vi "LvMPDC_SUB_ParseReplyString_Status.vi"(10 "status reply string":string="volume: 90\nrepeat: 0\nrandom: 0\nsingle: 0\nconsume: 1\nplaylist: 10\nplaylistlength: 6\nxfade: 0\nmixrampdb: 0.000000\nmixrampdelay: nan\nstate: play\nsong: 0\nsongid: 8\ntime: 48:264\nelapsed: 47.833\nbitrate: 128\naudio: 22050:24:1\nnextsong: 1\nnextsongid: 9\n") -> (2 "status":T1 {"elapsed" format="%<%H:%M:%S%3u>t"; "time" format="%<%H:%M:%S%3u>t"})   [LabVIEW 2012]
uses:
  LvMPDC_Typdef_status.ctl
panel:
  # "volume: 90\nrepeat: 0\nrandom: 0\nsingle: 0\nconsume: 1\nplaylist: 10\nplaylistlength: 6\nxfade: 0[sec]\nmixrampdb: 0.000000\nmixrampdelay: nan\nstate: play\nsong: 0\nsongid: 8\ntime: 48:264\nelapsed: 47.833\nbitrate: 128[kbps]\naudio: 22050:24:1\nnextsong: 1\nnextsongid: 9"
  # "volume: 90\nrepeat: 0\nrandom: 0\nsingle: 0\nconsume: 1\nplaylist: 16\nplaylistlength: 0\nxfade: 0\nmixrampdb: 0.000000[dB]\nmixrampdelay: nan[sec]\nstate: stop"
  # "audio: 22050:24:1 / samplerate:bits:channels"
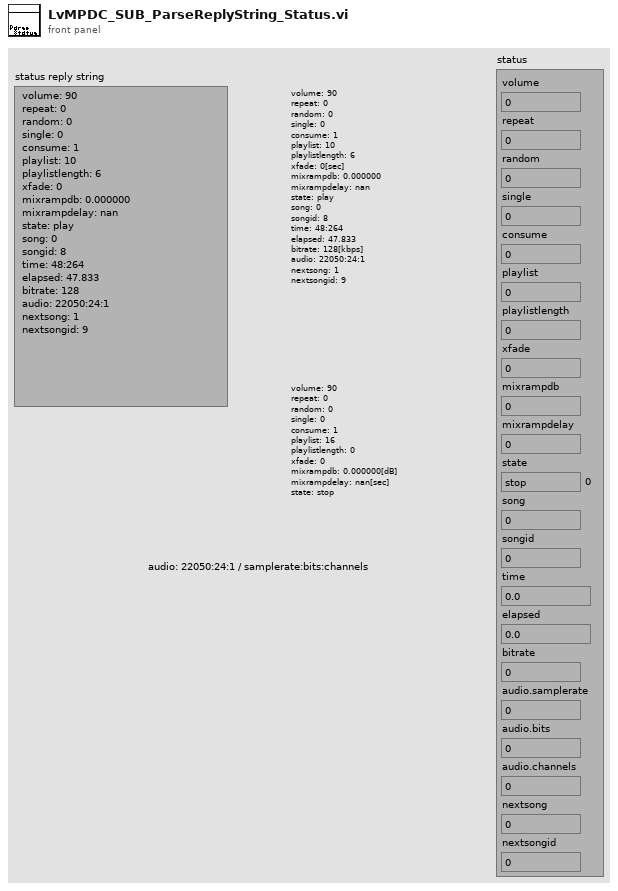
[diagram p1: front panel]
types:
  T1 = typedef "LvMPDC_Typdef_status.ctl" = cluster{"volume":i32, "repeat":i32, "random":i32, "single":i32, "consume":i32, "playlist":i32, "playlistlength":i32, "xfade":i32, "mixrampdb":dbl, "mixrampdelay":dbl, "state":enum16{"stop", "play", "pause"}, "song":i32, "songid":i32, "time":dbl, "elapsed":dbl, "bitrate":i32, "audio.samplerate":i32, "audio.bits":i32, "audio.channels":i32, "nextsong":i32, "nextsongid":i32}
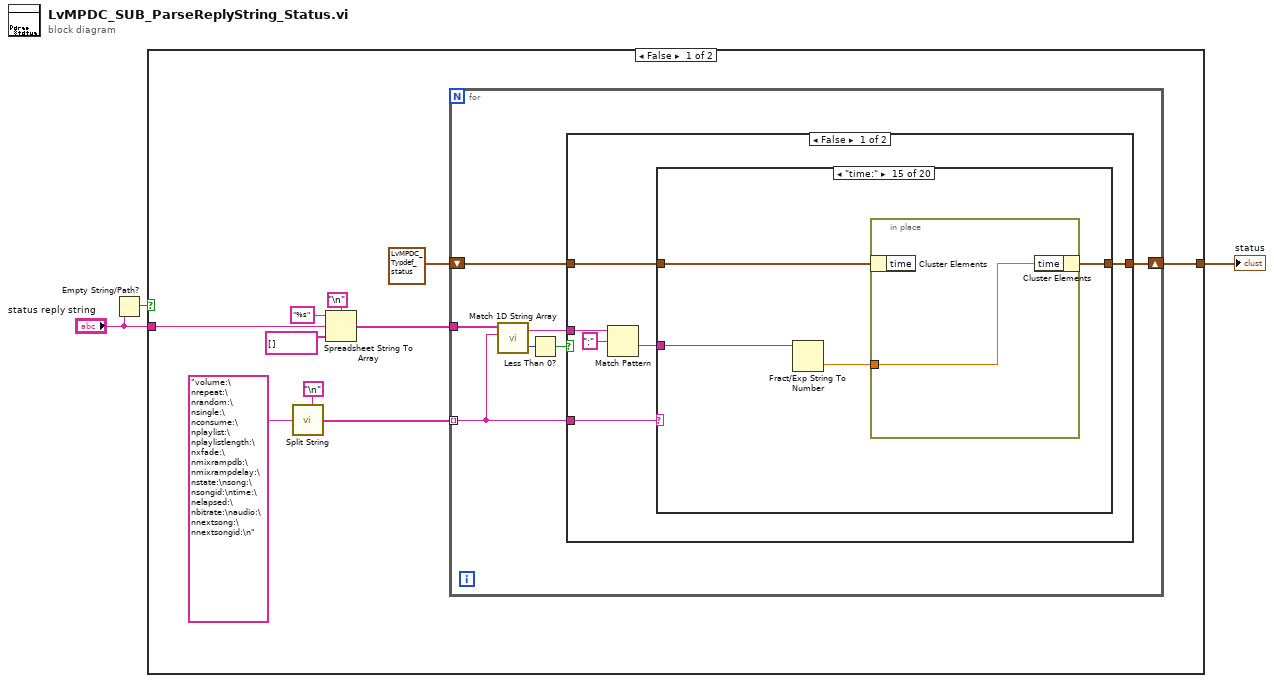
[diagram p0: block diagram]
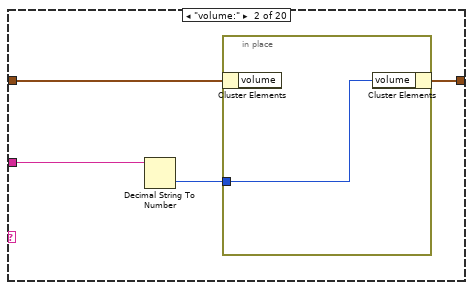
[diagram p3: hidden frame]
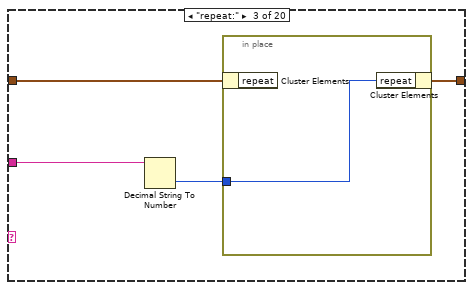
[diagram p4: hidden frame]
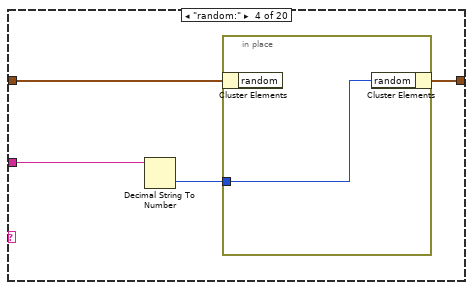
[diagram p5: hidden frame]
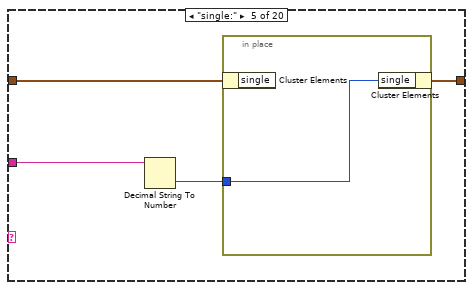
[diagram p6: hidden frame]
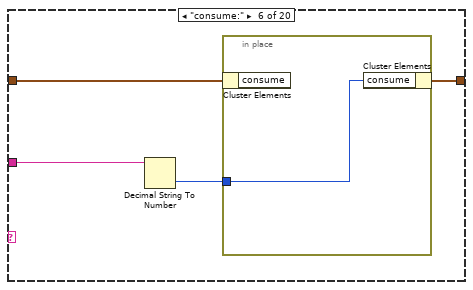
[diagram p7: hidden frame]
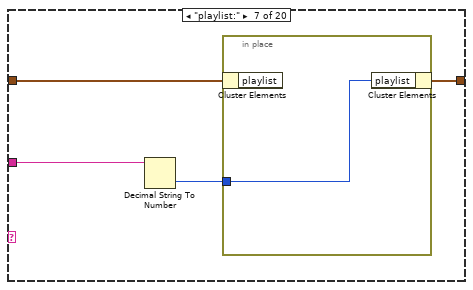
[diagram p8: hidden frame]
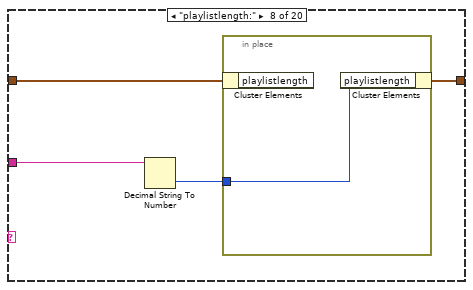
[diagram p9: hidden frame]
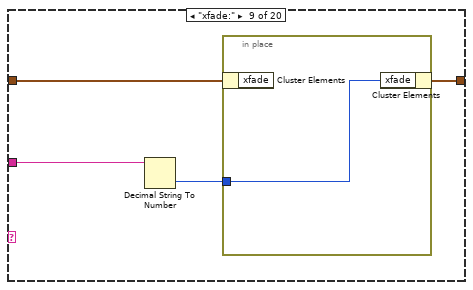
[diagram p10: hidden frame]
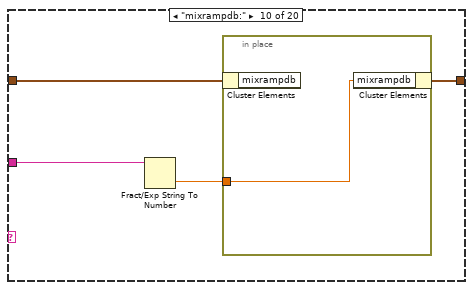
[diagram p11: hidden frame]
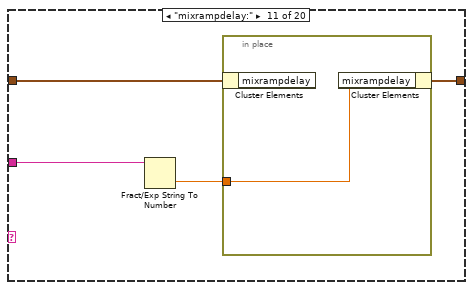
[diagram p12: hidden frame]
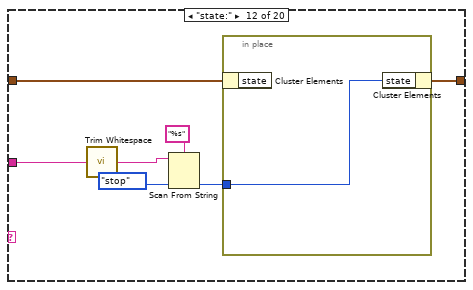
[diagram p13: hidden frame]
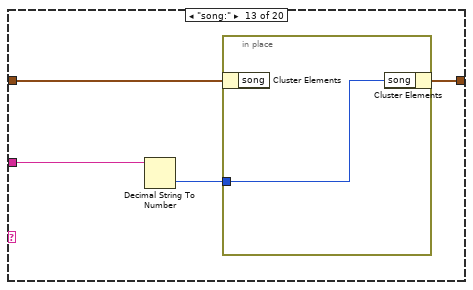
[diagram p14: hidden frame]
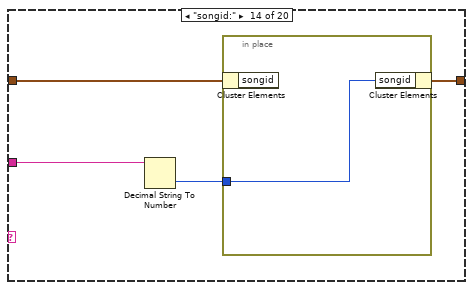
[diagram p15: hidden frame]
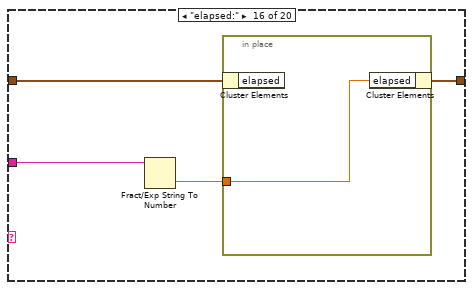
[diagram p16: hidden frame]
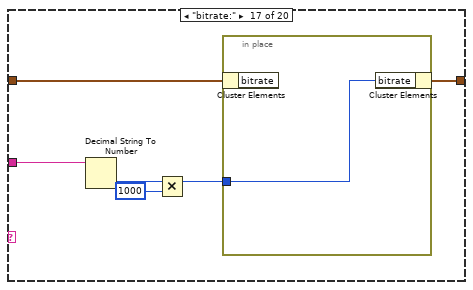
[diagram p17: hidden frame]
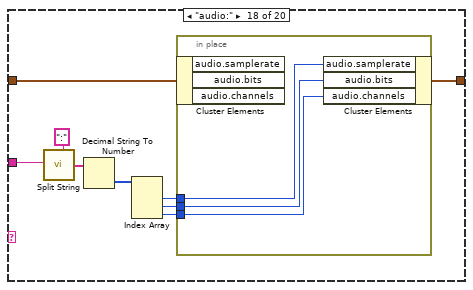
[diagram p18: hidden frame]
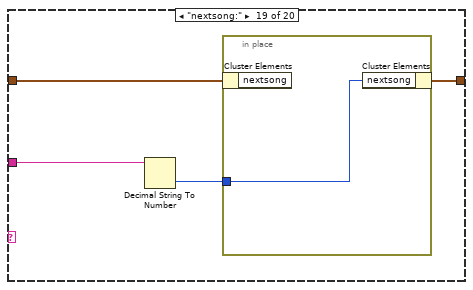
[diagram p19: hidden frame]
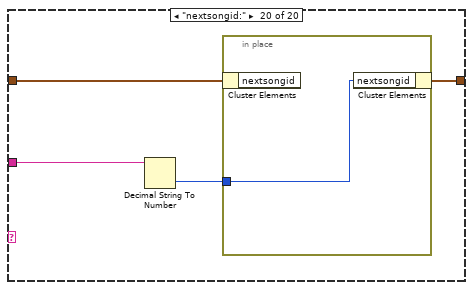
[diagram p20: hidden frame]
diagram:
  n1 = Empty String/Path?(string/path="status reply string") -> (empty?=w1:bool)
  n2 = case shown="FALSE" w1 {
    tunnel: "status reply string" -> [w10 _]
    tunnel: [w5 _] -> w3
    frame False {
      n3 = call <vilib>:"Split String.vi"("Split Pattern"="\n", "Input String"="volume:\nrepeat:\nrandom:\nsingle:\nconsume:\nplaylist:\nplaylistlength:\nxfade:\nmixrampdb:\nmixrampdelay:\nstate:\nsong:\nsongid:\ntime:\nelapsed:\nbitrate:\naudio:\nnextsong:\nnextsongid:\n") -> ("Split String"=w6:string[])  [unwired: 5 in]
      n4 = Spreadsheet String To Array(delimiter (Tab)="\n", format string="%s" ("形式文字列"), spreadsheet string=w10, array type (2D Dbl)=string[] []) -> (array=w9:string[])
      n5 = for {
        tunnel: w9 -> [w20]
        tunnel: w6 -> [w19] mode=indexing
        shift-right: [w14] -> w5
        shift-left: T1 {"volume"=0, "repeat"=0, "random"=0, "single"=0, "consume"=0, "playlist"=0, "playlistlength"=0, "xfade"=0, "mixrampdb"=0.0, "mixrampdelay"=0.0, "state"=enum."stop", "song"=0, "songid"=0, "time"=0.0, "elapsed"=0.0, "bitrate"=0, "audio.samplerate"=0, "audio.bits"=0, "audio.channels"=0, "nextsong"=0, "nextsongid"=0} ("status") -> [w15]
        n6 = call <vilib>:"Match 1D String Array.vi"("Pattern"=w19, "Strings"=w20) -> ("index of element"=w18:i32, "Match"=w17:string)  [unwired: 2 in]
        n7 = Less Than 0?(x=w18) -> (x < 0?=w16:bool)
        n8 = case shown="FALSE" w16 {
          tunnel: w19 -> [w26 _]
          tunnel: w17 -> [w22 _]
          tunnel: w15 -> [w25 w135]
          tunnel: [w24 w135] -> w14
          frame False {
            n9 = Match Pattern(string=w22, regular expression=":" ("正規表現")) -> (after substring=w21:string)  [unwired: 1 in, 3 out]
            n10 = case shown="\"time:\"" w26 {
              tunnel: w25 -> [w27 w31 w36 w41 w46 w51 w56 w61 w66 w71 w76 w84 w89 w94 w99 w104 w111 w121 w128 w133]
              tunnel: [w27 w30 w35 w40 w45 w50 w55 w60 w65 w70 w75 w83 w88 w93 w98 w103 w110 w120 w127 w132] -> w24
              tunnel: w21 -> [_ w29 w34 w39 w44 w49 w54 w59 w64 w69 w74 w82 w87 w92 w97 w102 w109 w119 w126 w131]
              frame Default {
              }
              frame "volume:" {
                n11 = Decimal String To Number(string=w29) -> (number=w28:i32)  [unwired: 2 in, 1 out]
                n12 = in-place {
                  in-place-border: w28 -> [w32]
                  n13 = in-place-cluster #1(w31) -> ()  [unwired: 1 out]
                  n14 = in-place-cluster #1("volume"=w32) -> (w30:T1)
                }
              }
              frame "repeat:" {
                n15 = Decimal String To Number(string=w34) -> (number=w33:i32)  [unwired: 2 in, 1 out]
                n16 = in-place {
                  in-place-border: w33 -> [w37]
                  n17 = in-place-cluster #2(w36) -> ()  [unwired: 1 out]
                  n18 = in-place-cluster #2("repeat"=w37) -> (w35:T1)
                }
              }
              frame "random:" {
                n19 = Decimal String To Number(string=w39) -> (number=w38:i32)  [unwired: 2 in, 1 out]
                n20 = in-place {
                  in-place-border: w38 -> [w42]
                  n21 = in-place-cluster #3(w41) -> ()  [unwired: 1 out]
                  n22 = in-place-cluster #3("random"=w42) -> (w40:T1)
                }
              }
              frame "single:" {
                n23 = Decimal String To Number(string=w44) -> (number=w43:i32)  [unwired: 2 in, 1 out]
                n24 = in-place {
                  in-place-border: w43 -> [w47]
                  n25 = in-place-cluster #4(w46) -> ()  [unwired: 1 out]
                  n26 = in-place-cluster #4("single"=w47) -> (w45:T1)
                }
              }
              frame "consume:" {
                n27 = Decimal String To Number(string=w49) -> (number=w48:i32)  [unwired: 2 in, 1 out]
                n28 = in-place {
                  in-place-border: w48 -> [w52]
                  n29 = in-place-cluster #5(w51) -> ()  [unwired: 1 out]
                  n30 = in-place-cluster #5("consume"=w52) -> (w50:T1)
                }
              }
              frame "playlist:" {
                n31 = Decimal String To Number(string=w54) -> (number=w53:i32)  [unwired: 2 in, 1 out]
                n32 = in-place {
                  in-place-border: w53 -> [w57]
                  n33 = in-place-cluster #6(w56) -> ()  [unwired: 1 out]
                  n34 = in-place-cluster #6("playlist"=w57) -> (w55:T1)
                }
              }
              frame "playlistlength:" {
                n35 = Decimal String To Number(string=w59) -> (number=w58:i32)  [unwired: 2 in, 1 out]
                n36 = in-place {
                  in-place-border: w58 -> [w62]
                  n37 = in-place-cluster #7(w61) -> ()  [unwired: 1 out]
                  n38 = in-place-cluster #7("playlistlength"=w62) -> (w60:T1)
                }
              }
              frame "xfade:" {
                n39 = Decimal String To Number(string=w64) -> (number=w63:i32)  [unwired: 2 in, 1 out]
                n40 = in-place {
                  in-place-border: w63 -> [w67]
                  n41 = in-place-cluster #8(w66) -> ()  [unwired: 1 out]
                  n42 = in-place-cluster #8("xfade"=w67) -> (w65:T1)
                }
              }
              frame "mixrampdb:" {
                n43 = Fract/Exp String To Number(string=w69) -> (number=w68:dbl)  [unwired: 3 in, 1 out]
                n44 = in-place {
                  in-place-border: w68 -> [w72]
                  n45 = in-place-cluster #9(w71) -> ()  [unwired: 1 out]
                  n46 = in-place-cluster #9("mixrampdb"=w72) -> (w70:T1)
                }
              }
              frame "mixrampdelay:" {
                n47 = Fract/Exp String To Number(string=w74) -> (number=w73:dbl)  [unwired: 3 in, 1 out]
                n48 = in-place {
                  in-place-border: w73 -> [w77]
                  n49 = in-place-cluster #10(w76) -> ()  [unwired: 1 out]
                  n50 = in-place-cluster #10("mixrampdelay"=w77) -> (w75:T1)
                }
              }
              frame "state:" {
                n51 = call <vilib>:"Trim Whitespace.vi"("string"=w82) -> ("trimmed string"=w78:string)  [unwired: 1 in]
                n52 = Scan From String(format string="%s" ("形式文字列"), input string=w78, default 1=enum16{"stop", "play", "pause"}."stop" ("state")) -> (output 1=w79:enum16{"stop", "play", "pause"})  [unwired: 2 in, 3 out]
                n53 = in-place {
                  in-place-border: w79 -> [w85]
                  n54 = in-place-cluster #11(w84) -> ()  [unwired: 1 out]
                  n55 = in-place-cluster #11("state"=w85) -> (w83:T1)
                }
              }
              frame "song:" {
                n56 = Decimal String To Number(string=w87) -> (number=w86:i32)  [unwired: 2 in, 1 out]
                n57 = in-place {
                  in-place-border: w86 -> [w90]
                  n58 = in-place-cluster #12(w89) -> ()  [unwired: 1 out]
                  n59 = in-place-cluster #12("song"=w90) -> (w88:T1)
                }
              }
              frame "songid:" {
                n60 = Decimal String To Number(string=w92) -> (number=w91:i32)  [unwired: 2 in, 1 out]
                n61 = in-place {
                  in-place-border: w91 -> [w95]
                  n62 = in-place-cluster #13(w94) -> ()  [unwired: 1 out]
                  n63 = in-place-cluster #13("songid"=w95) -> (w93:T1)
                }
              }
              frame "time:" {
                n64 = Fract/Exp String To Number(string=w97) -> (number=w96:dbl)  [unwired: 3 in, 1 out]
                n65 = in-place {
                  in-place-border: w96 -> [w100]
                  n66 = in-place-cluster #14(w99) -> ()  [unwired: 1 out]
                  n67 = in-place-cluster #14("time"=w100) -> (w98:T1)
                }
              }
              frame "elapsed:" {
                n68 = Fract/Exp String To Number(string=w102) -> (number=w101:dbl)  [unwired: 3 in, 1 out]
                n69 = in-place {
                  in-place-border: w101 -> [w105]
                  n70 = in-place-cluster #15(w104) -> ()  [unwired: 1 out]
                  n71 = in-place-cluster #15("elapsed"=w105) -> (w103:T1)
                }
              }
              frame "bitrate:" {
                n72 = Decimal String To Number(string=w109) -> (number=w108:i32)  [unwired: 2 in, 1 out]
                n73 = Multiply(x=w108, y=1000) -> (x*y=w107:i32)
                n74 = in-place {
                  in-place-border: w107 -> [w112]
                  n75 = in-place-cluster #16(w111) -> ()  [unwired: 1 out]
                  n76 = in-place-cluster #16("bitrate"=w112) -> (w110:T1)
                }
              }
              frame "audio:" {
                n77 = call <vilib>:"Split String.vi"("Split Pattern"=":", "Input String"=w119) -> ("Split String"=w117:string[])  [unwired: 5 in]
                n78 = Decimal String To Number(string=w117) -> (number=w116:i32[])  [unwired: 2 in, 1 out]
                n79 = Index Array(array=w116) -> (element #1=w115:i32, element #2=w114:i32, element #3=w113:i32)  [unwired: 3 in]
                n80 = in-place {
                  in-place-border: w115 -> [w124]
                  in-place-border: w114 -> [w123]
                  in-place-border: w113 -> [w122]
                  n81 = in-place-cluster #17(w121) -> ()  [unwired: 3 out]
                  n82 = in-place-cluster #17("audio.samplerate"=w124, "audio.bits"=w123, "audio.channels"=w122) -> (w120:T1)
                }
              }
              frame "nextsong:" {
                n83 = Decimal String To Number(string=w126) -> (number=w125:i32)  [unwired: 2 in, 1 out]
                n84 = in-place {
                  in-place-border: w125 -> [w129]
                  n85 = in-place-cluster #18(w128) -> ()  [unwired: 1 out]
                  n86 = in-place-cluster #18("nextsong"=w129) -> (w127:T1)
                }
              }
              frame "nextsongid:" {
                n87 = Decimal String To Number(string=w131) -> (number=w130:i32)  [unwired: 2 in, 1 out]
                n88 = in-place {
                  in-place-border: w130 -> [w134]
                  n89 = in-place-cluster #19(w133) -> ()  [unwired: 1 out]
                  n90 = in-place-cluster #19("nextsongid"=w134) -> (w132:T1)
                }
              }
            }
          }
          frame True {
          }
        }
      }
    }
    frame True {
    }
  }
  "status" <- w3
